vi "GlobalSettings.GetGroupName.vi"(11 "Name":string) -> (3 "Group":string)   [LabVIEW 2015, in "Fuel Injector Analysis Addon System Explorer.lvlib"]
uses:
  Fuel Injector Analysis Addon System Explorer.lvlib
  Shared/Constants.vi
  Shared/Fuel Injector Analysis Addon Shared.lvlib
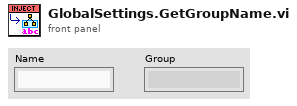
[diagram p1: front panel]
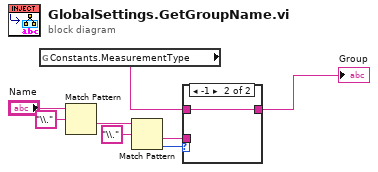
[diagram p0: block diagram]
diagram:
  n1 = global read "Constants.vi" "Constants.MeasurementType"() -> (w6:string)
  n2 = Match Pattern(string="Name", regular expression="\\.") -> (after substring=w4:string)  [unwired: 1 in, 3 out]
  n3 = Match Pattern(string=w4, regular expression="\\.") -> (after substring=w7:string, offset past match=w5:i32)  [unwired: 1 in, 2 out]
  n4 = case shown="-1" w5 {
    tunnel: w6 -> [_ w10]
    tunnel: [w9 w10] -> w8
    tunnel: w7 -> [w9 _]
    frame Default {
    }
    frame -1 {
    }
  }
  "Group" <- w8
